vi "Convert Array to CineStatus.vi"(10 "pCS array":u32[](array[numeric]), 11 "Numeric":i32=63) -> (3 "pCS out":T1[](array[typedef]))   [LabVIEW 2013, in "VRI.lvlib"]
uses:
  VRI.lvlib
  _Type Defs/PHCon CINESTATUS.ctl
panel:
  out "pCS":T1[](array[typedef])
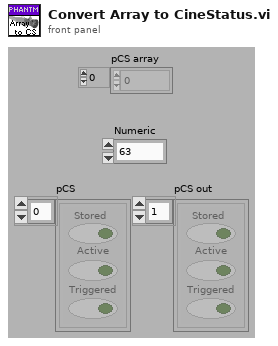
[diagram p1: front panel]
types:
  T1 = typedef "VRI.lvlib/PHCon CINESTATUS.ctl" = cluster{"Stored":bool, "Active":bool, "Triggered":bool}
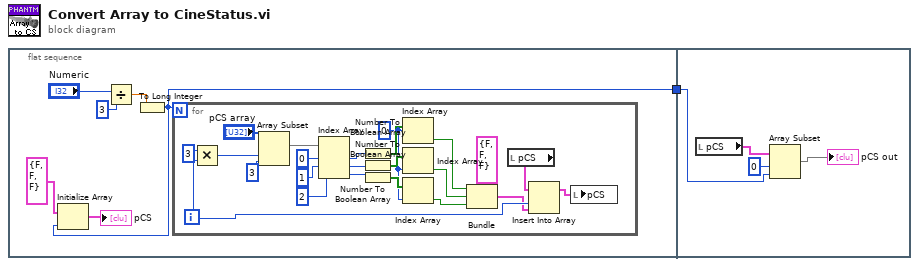
[diagram p0: block diagram]
diagram:
  n1 = flat-sequence {
    tunnel: [w2] -> w1
    tunnel: w1 -> [w32]
    frame #0 {
      n2 = Divide(x="Numeric", y=3) -> (x/y=w5:dbl)
      n3 = To Long Integer(number=w5) -> (32bit integer=w2:i32)
      n4 = Initialize Array(T1 {"Stored"=FALSE, "Active"=FALSE, "Triggered"=FALSE} ("CINESTATUS"), w2) -> (→"pCS":T1[])
      n5 = for {
        N: w2 -> [_]
        i -> [w13]
        w16 = 0 ("index")
        n6 = Multiply(x=3, y=w13) -> (x*y=w8:i32)
        n7 = Array Subset(array="pCS array", index=w8, length=3) -> (w28:u32[])
        n8 = Index Array(array=w28, index #1=0 ("index"), index #2=1 ("index"), index #3=2 ("index")) -> (element #1=w23:u32, element #2=w22:u32, element #3=w21:u32)
        n9 = Number To Boolean Array(number=w23) -> (Boolean array=w20:bool[])
        n10 = Number To Boolean Array(number=w22) -> (Boolean array=w18:bool[])
        n11 = Number To Boolean Array(number=w21) -> (Boolean array=w17:bool[])
        n12 = Index Array(array=w20, index=w16) -> (element=w19:bool)
        n13 = Index Array(array=w18, index=w16) -> (element=w15:bool)
        n14 = Index Array(array=w17, index=w16) -> (element=w14:bool)
        n15 = Bundle(cluster=T1 {"Stored"=FALSE, "Active"=FALSE, "Triggered"=FALSE} ("CINESTATUS"), "Stored"=w19, "Active"=w15, "Triggered"=w14) -> (w12:T1)
        n16 = local read "pCS"() -> (w11:T1[])
        n17 = Insert Into Array(array=w11, index=w13, new element=w12) -> (w9:T1[])
        n18 = local write "pCS"(w9) -> ()
      }
    }
    frame #1 {
      n19 = local read "pCS"() -> (w34:T1[])
      n20 = Array Subset(array=w34, index=0, length=w32) -> (→"pCS out":T1[])
    }
  }
